vi "dll.vi"() -> ()   [LabVIEW 2012]
uses:
  LabViewTestd.dll
panel:
  out "返回类型 2":dbl
  out "返回类型":dbl
  in  "b":dbl
  in  "a":dbl
  in  "nCols":i32
  in  "nRows":i32
  in  "pSrcPCCoord":dbl[][](array[numeric])
  # "a"
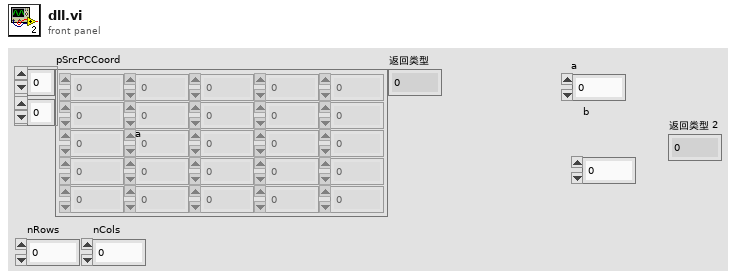
[diagram p1: front panel]
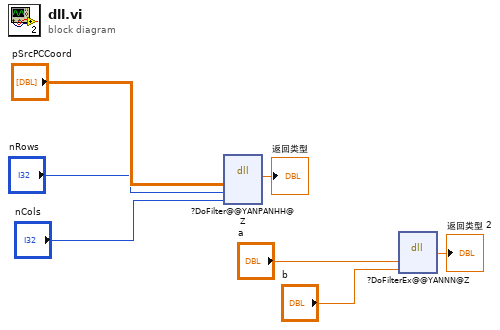
[diagram p0: block diagram]
diagram:
  n1 = dll-call lib="C:/Developer/labview/dll/LabViewTestd.dll" fn="?DoFilter@@YANPANHH@Z"("pSrcPCCoord"="pSrcPCCoord", "nRows"="nRows", "nCols"="nCols") -> ("返回类型"=→"返回类型":dbl)  [unwired: 6 in, 2 out]
  n2 = dll-call lib="C:/Developer/labview/dll/LabViewTestd.dll" fn="?DoFilterEx@@YANNN@Z"("a"="a", "b"="b") -> ("返回类型"=→"返回类型 2":dbl)  [unwired: 5 in, 2 out]
